vi "Insert Into Array (Single Numeric).vi"(9 "index":i32, 10 "Numeric":dbl, 11 "JSON Array in":refnum<class "JSON Array.lvclass">) -> (3 "JSON Array out":refnum<class "JSON Array.lvclass">)   [LabVIEW 2015, in "LVJSON.lvlib" / "JSON Array.lvclass"]
doc: "Inserts an element or subarray into a JSON array at the point you specify in index."
uses:
  JSON Array.lvclass
  Insert Into Array (Single).vi
  JSON Numeric/New JSON Numeric.vi
  JSON Helper/JSON Helper.lvclass
  JSON Numeric/JSON Numeric.lvclass
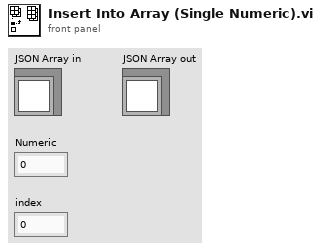
[diagram p1: front panel]
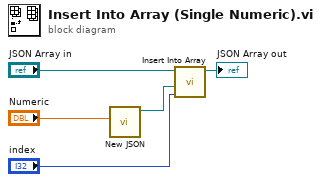
[diagram p0: block diagram]
diagram:
  n1 = call-poly "New JSON.vi"("value"="Numeric") -> ("JSON String out"=w2:refnum<class "JSON Numeric.lvclass">)  [unwired: 9 in, 1 out]
  n2 = call-poly "Insert Into Array.vi"("index"="index", "JSON Datatype"=w2, "JSON Array in"="JSON Array in") -> ("JSON Array out"=→"JSON Array out":refnum<class "JSON Array.lvclass">)  [unwired: 8 in]
